vi "Latch.vi"(11 "Latch In":bool) -> (3 "Latch Out":bool)   [LabVIEW 2012]
panel:
  in  "Default Value (false)":bool
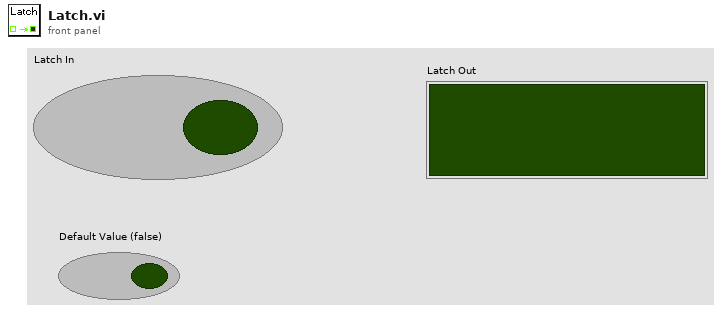
[diagram p1: front panel]
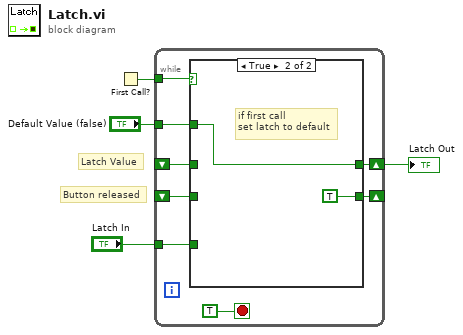
[diagram p0: block diagram]
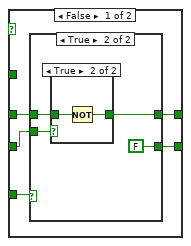
[diagram p2: hidden frame]
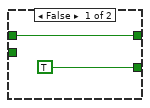
[diagram p3: hidden frame]
diagram:
  # "Latch Value"
  # "Button released"
  n1 = First Call?() -> (First Call?: T/F=w2:bool)
  n2 = while {
    tunnel: "Latch In" -> [w11]
    shift-right: [w10] -> _
    shift-left: _ -> [w7]
    shift-right: [w9] -> w3
    shift-left: _ -> [w8]
    tunnel: w2 -> [w6]
    tunnel: "Default Value (false)" -> [w5]
    stop <- TRUE stop-if-true
    n3 = case shown="True" w6 {
      tunnel: w11 -> [w17 _]
      tunnel: [w16 TRUE] -> w10
      tunnel: [w15 w27] -> w9
      tunnel: w8 -> [w14 _]
      tunnel: w7 -> [w13 _]
      tunnel: w5 -> [_ w27]
      frame False {
        n4 = case shown="True" w17 {
          tunnel: [TRUE FALSE] -> w16
          tunnel: [w18 w22] -> w15
          tunnel: w14 -> [w18 w21]
          tunnel: w13 -> [_ w20]
          frame False {
          }
          frame True {
            n5 = case shown="True" w20 {
              tunnel: [w24 w26] -> w22
              tunnel: w21 -> [w24 w25]
              frame False {
              }
              frame True {
                n6 = Not(x=w25) -> (.not. x?=w26:bool)
              }
            }
          }
        }
      }
      frame True {
        # "if first call\nset latch to default"
      }
    }
  }
  "Latch Out" <- w3
